vi "Projeto_final.vi"() -> ()   [LabVIEW 2019]
uses:
  <vilib>/myRIO/Instrument Drivers/Onboard IO/AI/typedefs/AI Reference.ctl
  <vilib>/myRIO/Common/Instrument Driver Framework/Utilities/typedefs/myRIO Generic Hardware Reference.ctl
  <vilib>/myRIO/Common/Instrument Driver Framework/Utilities/typedefs/Hardware Version Enum.ctl
  <vilib>/myRIO/Common/Instrument Driver Framework/Utilities/typedefs/myRIO v1.0 Reference.ctl
  <vilib>/myRIO/Common/Instrument Driver Framework/Utilities/typedefs/Generic FPGA Reference.ctl
  <vilib>/myRIO/Common/Instrument Driver Framework/myRIO v1.0/AI/typedefs/AI Channels List.ctl
  <vilib>/myRIO/Common/Instrument Driver Framework/myRIO v1.0/AI/typedefs/AI Channels Enum.ctl
  <vilib>/myRIO/Common/Instrument Driver Framework/Utilities/typedefs/Analog Scaling Constants List.ctl
  <vilib>/myRIO/Common/Instrument Driver Framework/Utilities/typedefs/Analog Scaling Constants.ctl
  <vilib>/userDefined/High Color/nirio_resource_hc.ctl
  <vilib>/myRIO/Common/Instrument Driver Framework/Utilities/vis/Is FPGA Ref Available.vi
  <vilib>/myRIO/Common/Instrument Driver Framework/myRIO v1.0/AI/vis/myRIO v1.1 Open AI.vi
  <vilib>/myRIO/Instrument Drivers/Onboard IO/AI/vis/Read.vi
  <vilib>/myRIO/Common/Instrument Driver Framework/Utilities/vis/Validate Channels.vi
  <vilib>/myRIO/Common/Instrument Driver Framework/myRIO v1.0/AI/vis/myRIO v1.0 Reserve AI.vi
  <vilib>/myRIO/Common/Instrument Driver Framework/myRIO v1.0/AI/vis/myRIO v1.0 Build MUX Configuration AI.vi
  <vilib>/myRIO/Common/Instrument Driver Framework/myRIO v1.0/Resource Manager/vis/myRIO v1.0 Reserve Channel List.vi
  <vilib>/myRIO/Common/Instrument Driver Framework/myRIO v1.0/Resource Manager/vis/myRIO v1.0 Reserve Channel.vi
  <vilib>/myRIO/Common/Instrument Driver Framework/myRIO v1.0/Resource Manager/vis/myRIO v1.0 Unreserve Channel.vi
  <vilib>/myRIO/Common/Instrument Driver Framework/myRIO v1.0/Resource Manager/vis/myRIO v1.0 Build Mutex Name.vi
  <vilib>/Utility/VariantDataType/GetNumericInfo.vi
  <vilib>/Utility/error.llb/Error Cluster From Error Code.vi
  <vilib>/myRIO/Common/Instrument Driver Framework/myRIO v1.0/myRIO v1.1 Open.vi
  <vilib>/myRIO/Common/Instrument Driver Framework/myRIO v1.0/AI/vis/myRIO v1.0 Get Scaling Constants AI.vi
  <vilib>/myRIO/Common/Instrument Driver Framework/Utilities/vis/IO Manager.vi
  <vilib>/myRIO/Common/Instrument Driver Framework/Utilities/vis/Configuration Manager.vi
  <vilib>/myRIO/Common/Instrument Driver Framework/myRIO v1.0/myRIO v1.0 Close.vi
  <vilib>/myRIO/Common/Instrument Driver Framework/myRIO v1.0/AI/vis/myRIO v1.0 Read AI.vi
  <vilib>/myRIO/Express VI/Onboard IO/AI/AI Express VI.xnode
  <vilib>/myRIO/Instrument Drivers/Onboard IO/AI/vis/myRIO AI Open.xnode
  <vilib>/myRIO/Instrument Drivers/Onboard IO/AI/AI.lvlib
panel:
  out "ERROR":bool
  in  "POWER":bool
  in  "SET TEMP":dbl(slide) scale=0.0..50.0
  out "THERMOMETER":dbl(slide) scale=0.0..100.0
  in  "?":bool
  out "?":bool
  # "Thermostat"
  # "COOL"
  # "ON"
  # "OF"
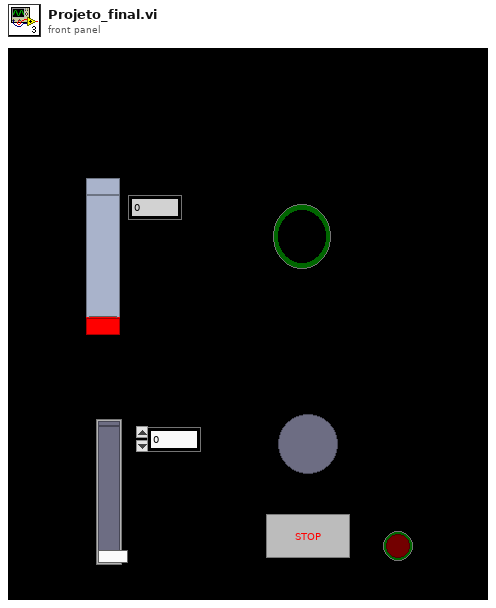
[diagram p1: front panel]
types:
  T1 = typedef "AI.lvlib/AI Reference.ctl" = cluster{"myRIO Reference":T2, "AI Channels List":T6, "AI Scaling Constants List":T8}
  T2 = typedef "myRIO Generic Hardware Reference.ctl" = cluster{"myRIO Model":T3, "myRIO Hardware Reference":T4}
  T3 = typedef "Hardware Version Enum.ctl" = enum16{"Unknown", "myRIO-1900", "myRIO-1950", "roboRIO", "NI ELVIS RIO CM", "ELVIS III"}
  T4 = typedef "myRIO v1.0 Reference.ctl" = cluster{"Generic FPGA Reference":T5, "Allow multiple opens":bool}
  T5 = typedef "Generic FPGA Reference.ctl" = refnum<k20>
  T6 = typedef "AI Channels List.ctl" = T7[]
  T7 = typedef "AI Channels Enum.ctl" = enum16{"Not Connected", "AudioIn/Left", "AudioIn/Right", "C/AI0", "C/AI1", "A/AI0", "A/AI1", "A/AI2", "A/AI3", "A/AI4", "A/AI5", "A/AI6", "A/AI7", "B/AI0", "B/AI1", "B/AI2", "B/AI3", "B/AI4", "B/AI5", "B/AI6", "B/AI7", "AI/AI0", "AI/AI1", "AI/AI2", "AI/AI3", "A/AI0 (DIFF)", "A/AI1 (DIFF)", "A/AI2 (DIFF)", "A/AI3 (DIFF)", "B/AI0 (DIFF)", "B/AI1 (DIFF)", "B/AI2 (DIFF)", "B/AI3 (DIFF)"}
  T8 = typedef "Analog Scaling Constants List.ctl" = T9[]
  T9 = typedef "Analog Scaling Constants.ctl" = cluster{"LSB Weight (Volts)":dbl, "Offset (Volts)":dbl, "Signed?":bool}
  T10 = typedef "nirio_resource_hc.ctl" = tag
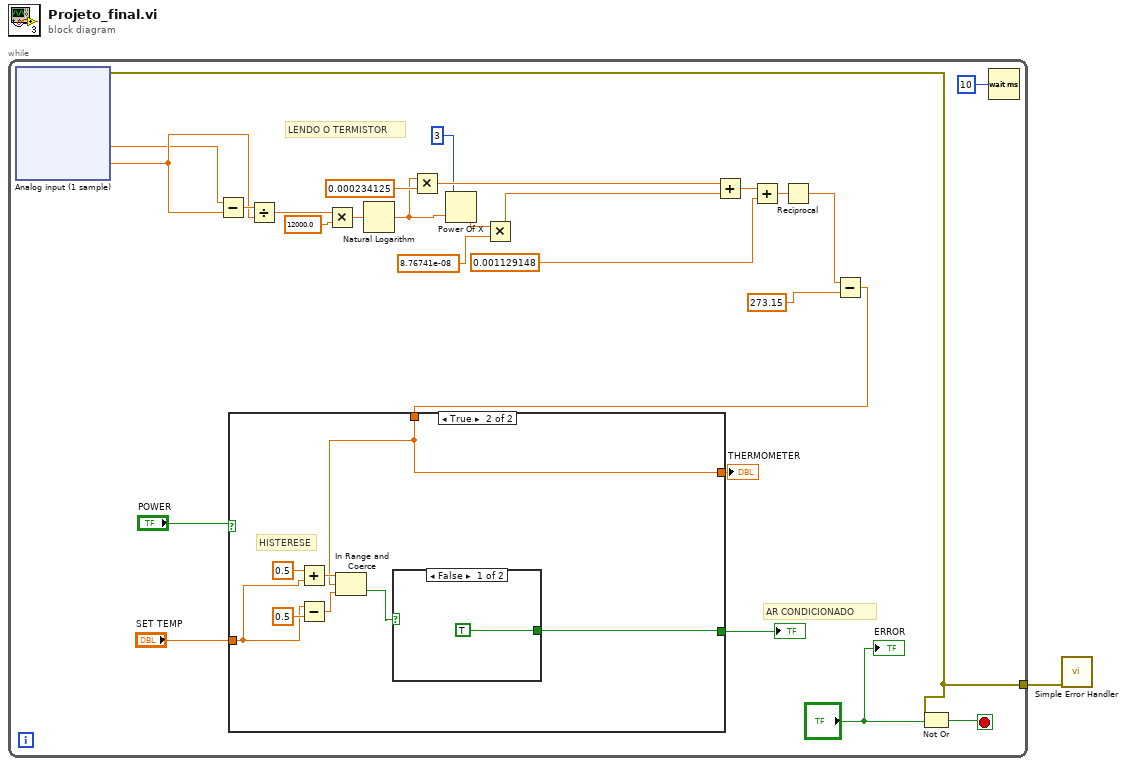
[diagram p0: block diagram]
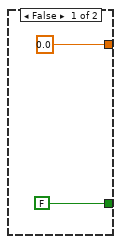
[diagram p2: hidden frame]
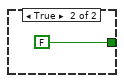
[diagram p3: hidden frame]
diagram:
  n1 = while {
    tunnel: [w22] -> w1
    stop <- w23 stop-if-true
    # "LENDO O TERMISTOR"
    # "AR CONDICIONADO"
    n2 = xnode "Analog input (1 sample)"() -> ("A/AI0 (Pin 3)"=w2:dbl, "A/AI1 (Pin 5)"=w3:dbl, "error out"=w22:errorcluster)  [unwired: 1 in]
    n3 = Subtract(x=w2, y=w3) -> (x-y=w27:dbl)
    n4 = Divide(x=w27, y=w3) -> (x/y=w26:dbl)
    n5 = Multiply(x=w26, y=12000.0) -> (x*y=w20:dbl)
    n6 = Natural Logarithm(1:w20) -> (0:w8:dbl)
    n7 = Multiply(x=w8, y=0.000234125) -> (x*y=w18:dbl)
    n8 = Power Of X(1:w8, 2:3) -> (0:w16:dbl)
    n9 = Multiply(x=w16, y=8.76741e-08) -> (x*y=w17:dbl)
    n10 = Add(x=w18, y=w17) -> (x+y=w14:dbl)
    n11 = Add(x=w14, y=0.001129148) -> (x+y=w12:dbl)
    n12 = Reciprocal(x=w12) -> (1/x=w6:dbl)
    n13 = Subtract(x=w6, y=273.15) -> (x-y=w4:dbl)
    n14 = case shown="True" "POWER" {
      tunnel: [0.0 w33] -> w24
      tunnel: "SET TEMP" -> [_ w36]
      tunnel: w4 -> [_ w33]
      tunnel: [FALSE w31] -> w11
      frame False {
      }
      frame True {
        # "HISTERESE"
        n15 = Add(x=0.5, y=w36) -> (x+y=w35:dbl)
        n16 = Subtract(x=w36, y=0.5) -> (x-y=w34:dbl)
        n17 = In Range and Coerce(upper limit=w35, x=w33, lower limit=w34) -> (In Range?=w32:bool)  [unwired: 1 out]
        n18 = case shown="False" w32 {
          tunnel: [TRUE FALSE] -> w31
          frame False {
          }
          frame True {
          }
        }
      }
    }
    "THERMOMETER" <- w24
    "?" <- w11
    n19 = Not Or(1:"?", 2:w22) -> (0:w23:bool)
    n20 = Wait (ms)(milliseconds to wait=10) -> ()  [unwired: 1 out]
    "ERROR" <- "?"
  }
  n21 = call <vilib>:"Simple Error Handler.vi"("error in (no error)"=w1) -> ()  [unwired: 4 in, 5 out]
